vi "JKISM++ Module Turns Invalid.vi"(3 "JKISM Name":string) -> (1 "Turn Invalid(Exit)?":bool)   [LabVIEW 2014, in "JKI State Machine++.lvlib"]
doc: "检查JKISM是否已经退出。通常用于和JKISM并行的功能循环，这些功能循环和 JKISM 一起完成完整模块功能。 本VI用于并行循环的退出条件。\n\n<b>Inputs:</b>\n - <b>JKISM Name</b>: 模块名称\n\n<b>Outputs:</b>\n - <b>Turn Invalid(Exit)?</b>: 是否已经退出"
uses:
  JKI State Machine++.lvlib
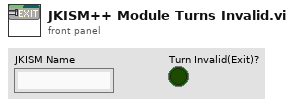
[diagram p1: front panel]
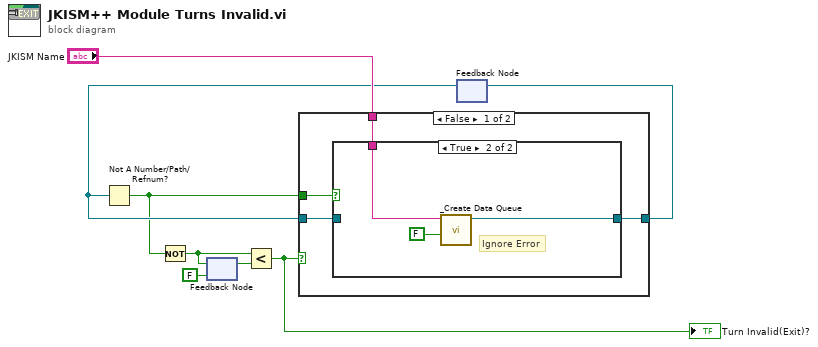
[diagram p0: block diagram]
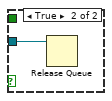
[diagram p3: hidden frame]
diagram:
  n1 = feedback #1(FALSE) -> (w5:bool)
  n2 = feedback #2() -> (w7:refnum<queue>)  [unwired: 1 in]
  n3 = Not A Number/Path/Refnum?(number/path/refnum=w7) -> (NaN/Path/Refnum?=w2:bool)
  n4 = Not(x=w2) -> (.not. x?=w6:bool)
  n5 = feedback-in #1(w6) -> ()
  n6 = Less?(x=w6, y=w5) -> (x < y?=w1:bool)
  "Turn Invalid(Exit)?" <- w1
  n7 = case shown="False" w1 {
    tunnel: "JKISM Name" -> [w12 _]
    tunnel: w7 -> [w11 w17]
    tunnel: [w10 _] -> w3
    tunnel: w2 -> [w9 _]
    frame False {
      n8 = case shown="True" w9 {
        tunnel: w12 -> [_ w16]
        tunnel: [w13 w14] -> w10
        tunnel: w11 -> [w13 _]
        frame False {
        }
        frame True {
          # "Ignore Error"
          n9 = call "_Create Data Queue.vi"("create if not found? (T)"=FALSE, "Name"=w16) -> ("Queue out"=w14:refnum<queue>)  [unwired: 7 in, 2 out]
        }
      }
    }
    frame True {
      n10 = Release Queue(queue=w17) -> ()  [unwired: 2 in, 3 out]
    }
  }
  n11 = feedback-in #2(w3) -> ()
